vi "MouseclickMultipassChannel.vi"(10 "error in (no error)":errorcluster) -> (2 "error out":errorcluster)   [LabVIEW 2014]
panel:
  in  "AutoItX3Lib.IAutoItX3":refnum<k7>
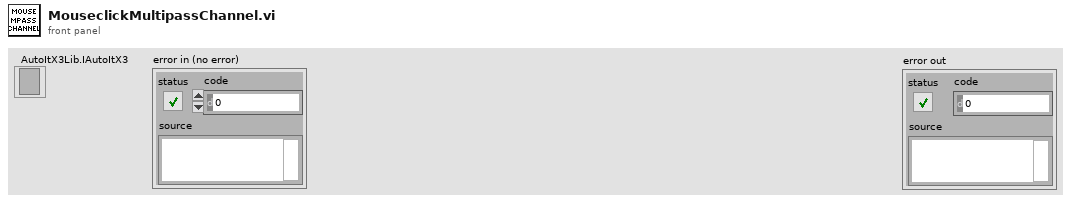
[diagram p1: front panel]
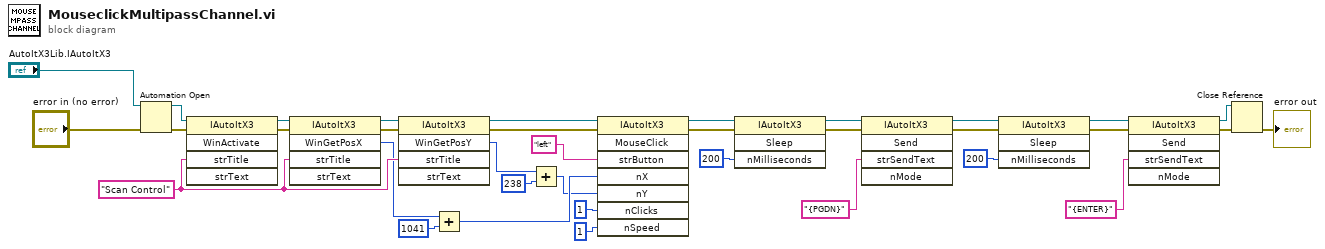
[diagram p0: block diagram]
diagram:
  w25 = "Scan Control" ("strTitle")
  n1 = Automation Open(error in (no error)="error in (no error)", Automation Refnum="AutoItX3Lib.IAutoItX3") -> (Automation Refnum=w31:refnum<k7>, error out=w30:errorcluster)  [unwired: 2 in]
  n2 = invoke class="IAutoItX3" method="WinActivate"(reference=w31, error in=w30, "strTitle"=w25) -> (reference out=w29:refnum<k7>, error out=w28:errorcluster)  [unwired: 2 in, 3 out]
  n3 = invoke class="IAutoItX3" method="WinGetPosX"(reference=w29, error in=w28, "strTitle"=w25) -> (reference out=w27:refnum<k7>, error out=w26:errorcluster, "WinGetPosX"=w23:i32)  [unwired: 2 in, 2 out]
  n4 = invoke class="IAutoItX3" method="WinGetPosY"(reference=w27, error in=w26, "strTitle"=w25) -> (reference out=w17:refnum<k7>, error out=w16:errorcluster, "WinGetPosY"=w24:i32)  [unwired: 2 in, 2 out]
  n5 = Add(x=w23, y=1041) -> (x+y=w19:i32)
  n6 = Add(x=w24, y=238) -> (x+y=w18:i32)
  n7 = invoke class="IAutoItX3" method="MouseClick"(reference=w17, error in=w16, "strButton"="left", "nX"=w19, "nY"=w18, "nClicks"=1, "nSpeed"=1) -> (reference out=w33:refnum<k7>, error out=w32:errorcluster)  [unwired: 1 in, 6 out]
  n8 = invoke class="IAutoItX3" method="Sleep"(reference=w33, error in=w32, "nMilliseconds"=200) -> (reference out=w13:refnum<k7>, error out=w12:errorcluster)  [unwired: 1 in, 2 out]
  n9 = invoke class="IAutoItX3" method="Send"(reference=w13, error in=w12, "strSendText"="{PGDN}") -> (reference out=w11:refnum<k7>, error out=w10:errorcluster)  [unwired: 2 in, 3 out]
  n10 = invoke class="IAutoItX3" method="Sleep"(reference=w11, error in=w10, "nMilliseconds"=200) -> (reference out=w9:refnum<k7>, error out=w8:errorcluster)  [unwired: 1 in, 2 out]
  n11 = invoke class="IAutoItX3" method="Send"(reference=w9, error in=w8, "strSendText"="{ENTER}") -> (reference out=w7:refnum<k7>, error out=w6:errorcluster)  [unwired: 2 in, 3 out]
  n12 = Close Reference(reference=w7, error in (no error)=w6) -> (error out=→"error out":errorcluster)
